vi "writeToXML.vi"(8 "error in (no error)":errorcluster, 10 "ClassLabel":string, 11 "OffsetDef in":refnum<class "OffsetDef.lvclass">) -> (0 "error out":errorcluster, 2 "XML out":string, 3 "OffsetDef out":refnum<class "OffsetDef.lvclass">)   [LabVIEW 2014, in "TCSDataDefinitions.lvlib" / "TCSCommand.lvlib" / "OffsetCommands.lvlib" / "OffsetDef.lvclass"]
uses:
  OffsetDef.lvclass
  <userlib>/Common/UnitsAndXML/FlattenItemWithUnitToXML/FlattenTimeToXML/TimeUnit.ctl
  <userlib>/Common/UnitsAndXML/FlattenItemWithUnitToXML/FlattenPlaneAngleToXML/PlaneAngleUnit.ctl
  OffsetDef.lvclass/OffsetDef.ctl
  <userlib>/Common/UnitsAndXML/UnitsAndXML.lvlib
  <userlib>/Common/XML/XMLGenerator/XMLGenerator.lvclass
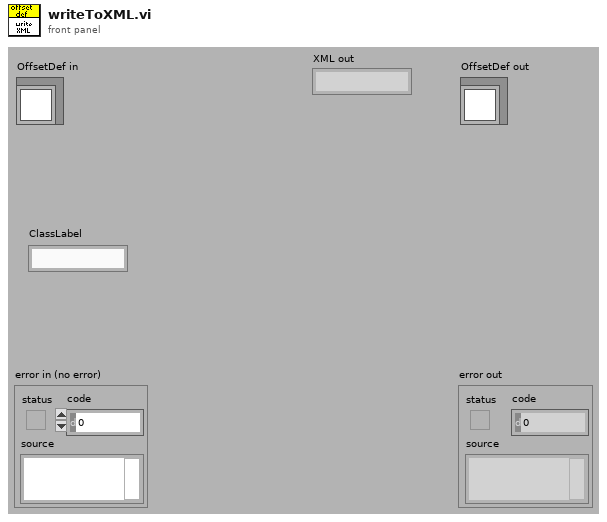
[diagram p1: front panel]
types:
  T1 = typedef "UnitsAndXML.lvlib/PlaneAngleUnit.ctl" = enum16{"rad", "deg", "'", "\""}
  T2 = typedef "UnitsAndXML.lvlib/TimeUnit.ctl" = enum16{"s", "d", "h", "min", "a"}
  T3 = typedef "TCSDataDefinitions.lvlib/TCSCommand.lvlib/OffsetCommands.lvlib/Num1Types.ctl" = enum16{"User", "Handset"}
  T4 = typedef "TCSDataDefinitions.lvlib/TCSCommand.lvlib/OffsetCommands.lvlib/OffsetType.ctl" = enum16{"SIMPLE", "TPLANE", "PA"}
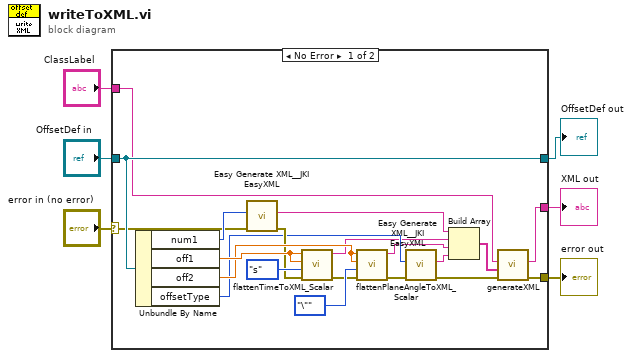
[diagram p0: block diagram]
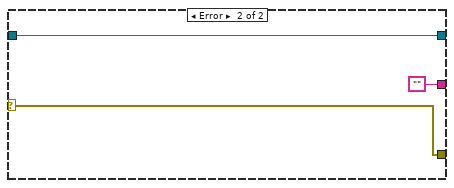
[diagram p2: hidden frame]
diagram:
  n1 = case shown="No Error" "error in (no error)" {
    selector: "error in (no error)" -> [w10 w29]
    tunnel: [w9 w29] -> w5
    tunnel: [w26 w28] -> w3
    tunnel: "OffsetDef in" -> [w26 w28]
    tunnel: "ClassLabel" -> [w8 _]
    tunnel: [w7 ""] -> w1
    frame No Error {
      n2 = Unbundle By Name(w26) -> ("num1"=w20:T3, "off1"=w25:dbl[unit], "off2"=w23:dbl[unit], "offsetType"=w18:T4)
      n3 = call <vilib>:"Easy Generate XML__JKI EasyXML.vi"("error in (no error)"=w10, "LabVIEW Data"=w20) -> ("error out"=w19:errorcluster, "XML String"=w15:string)  [unwired: 8 in]
      n4 = call <userlib>:"flattenTimeToXML_Scalar.vi"("error in (no error)"=w19, "timeUnitInXML"=TimeUnit."s", "timeAgain"=w25, "time"=w25) -> ("error out"=w21:errorcluster, "xmlString"=w14:string)  [unwired: 6 in]
      n5 = call <userlib>:"flattenPlaneAngleToXML_Scalar.vi"("error in (no error)"=w21, "planeAngleUnitInXML"=PlaneAngleUnit."\"", "planeAngleAgain"=w23, "planeAngle"=w23) -> ("error out"=w17:errorcluster, "xmlString"=w13:string)  [unwired: 6 in]
      n6 = call <vilib>:"Easy Generate XML__JKI EasyXML.vi"("error in (no error)"=w17, "LabVIEW Data"=w18) -> ("error out"=w11:errorcluster, "XML String"=w12:string)  [unwired: 8 in]
      n7 = Build Array(w15, w14, w13, w12) -> (w16:string[])
      n8 = call <userlib>:"generateXML.vi"("error in"=w11, "childrenXML"=w16, "elementName"=w8) -> ("error out"=w9:errorcluster, "XML out"=w7:string)  [unwired: 6 in, 1 out]
    }
    frame Error {
    }
  }
  "error out" <- w5
  "OffsetDef out" <- w3
  "XML out" <- w1
